vi "libdaq_pwm_config.vi"(0 "error in (no error)":errorcluster, 1 "device_name":string, 2 "module_name":string) -> (14 "error out":errorcluster, 15 "device_name":string, 16 "module_name":string)   [LabVIEW 2010, in "libdaqVI.lvlib"]
uses:
  libdaqVI.lvlib
  dll/daqlib.dll
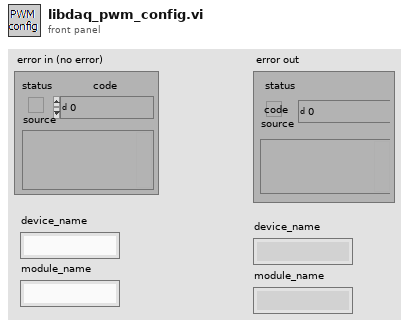
[diagram p1: front panel]
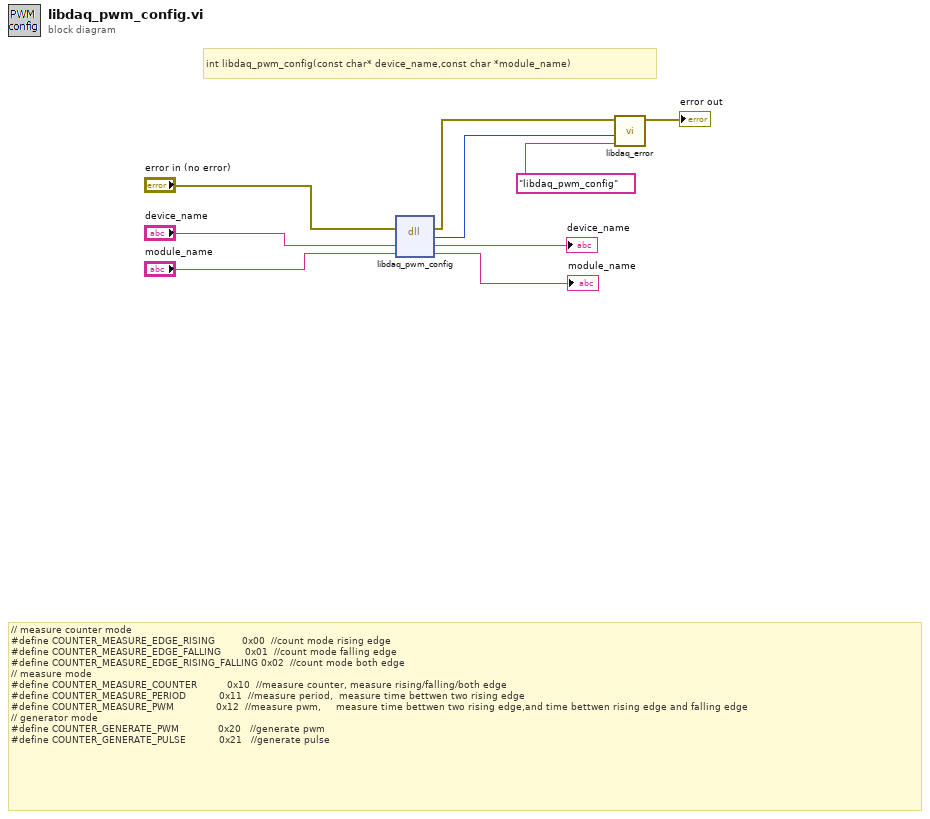
[diagram p0: block diagram]
diagram:
  # "// measure counter mode\n#define COUNTER_MEASURE_EDGE_RISING         0x00  //count mode rising edge\n#define COUNTER_MEASURE_EDGE_FALLING        0x01  //count mode falling edge\n#define COUNTER_MEASURE_EDGE_RISING_FALLING 0x02  //count mode both edge\n// measure mode\n#define COUNTER_MEASURE_COUNTER          0x10  //measure counter, measure rising/falling/both edge\n#define COUNTER_MEASURE_PERIOD           0x11  //measure period,  measure time bettwen two rising edge\n#define COUNTER_MEASURE_PWM              0x12  //measure pwm,     measure time bettwen two rising edge,and time bettwen rising edge and falling edge\n// generator mode\n#define COUNTER_GENERATE_PWM             0x20   //generate pwm\n#define COUNTER_GENERATE_PULSE           0x21   //generate pulse"
  # "int libdaq_pwm_config(const char* device_name,const char *module_name)"
  n1 = dll-call lib="E:/Product/Example/DAQ-USB3212/Labview/labview_2010/libdaqVI/dll/daqlib.dll" fn="libdaq_pwm_config"(error in="error in (no error)", "device_name"="device_name", "module_name"="module_name") -> (error out=w4:errorcluster, "return type"=w2:i32, "device_name"=→"device_name":string, "module_name"=→"module_name":string)  [unwired: 2 in, 1 out]
  n2 = call "libdaq_error.vi"("error source"="libdaq_pwm_config", "error code"=w2, "错误输入（无错误）"=w4) -> ("错误输出"=→"error out":errorcluster)  [unwired: 8 in]
